vi "MoAgSy_AgentBase.appendData2Variant.vi"(0 "init":variant, 1 "Agent name":string, 2 "journey":string[](array[string]), 3 "Command names":string[](array[string]), 5 "error in":errorcluster, 7 "standard Visitor timeout in ms":i32, 9 "standard visitor":refnum<class "MoAgSy_Visitor.lvclass">) -> (14 "dup init":variant, 19 "error out":errorcluster)   [LabVIEW 2009, in "MoAgSy_Base.lvlib" / "MoAgSy_AgentBase.lvclass"]
doc: "Empty Agent Name:\nKey ID is set as Agent Name"
uses:
  MoAgSy_AgentBase.lvclass
  Visitors/MoAgSy_Visitor/MoAgSy_Visitor.lvclass
  MoAgSy_GPG/MoAgSy_GPG.lvclass
  MoAgSy_Factory/MoAgSy_Factory.lvclass
  HGF_BaseClasses/HGF_Factory/HGF_Factory.lvclass
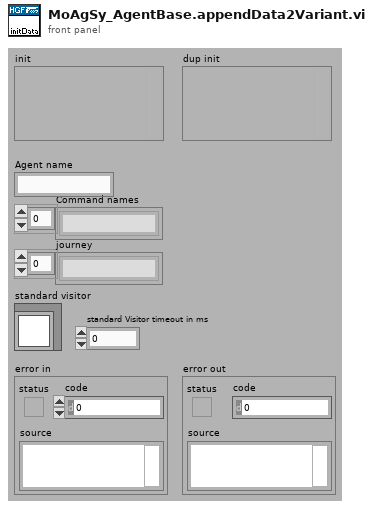
[diagram p1: front panel]
types:
  T1 = cluster{"standard visitor":refnum<class "MoAgSy_Visitor.lvclass">, "standard Visitor timeout in ms":i32}
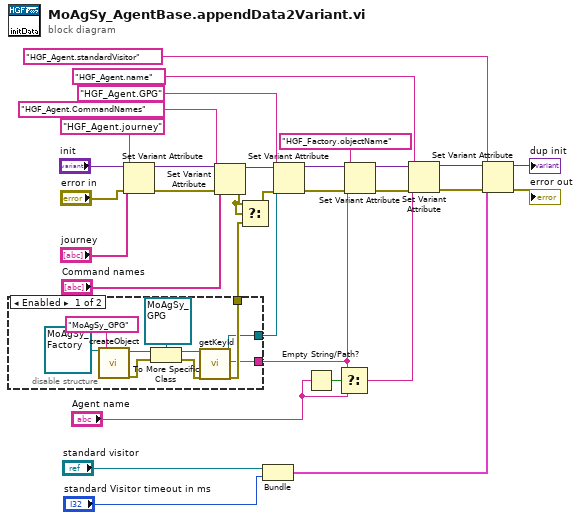
[diagram p0: block diagram]
diagram:
  n1 = disable-structure shown="Enabled" {
    disable-tunnel: [w34 _] -> w22
    disable-tunnel: [w33 _] -> w21
    disable-tunnel: [w32 _] -> w12
    frame #0 {
      n2 = call "createObject.vi"("HGF_Factory"=refnum<class "MoAgSy_Factory.lvclass"> refnum ("MoAgSy.lvlib:MoAgSy_Factory.lvclass"), "className"="MoAgSy_GPG") -> ("HGF_Object"=w39:refnum<class "HGF_Factory.lvclass">, "error out"=w40:errorcluster)  [unwired: 3 in, 13 out]
      n3 = To More Specific Class(target class=refnum<class "MoAgSy_GPG.lvclass"> refnum ("MoAgSy.lvlib:MoAgSy_GPG.lvclass"), reference=w39, error in=w40) -> (specific class reference=w36:refnum<class "MoAgSy_GPG.lvclass">, error out=w35:errorcluster)
      n4 = call-dynamic "getKeyId.vi"("HGF_GPG.lvclass in"=w36, "error in (no error)"=w35) -> ("HGF_GPG.lvclass out"=w33:refnum<class "MoAgSy_GPG.lvclass">, "Key-ID"=w32:string, "error out"=w34:errorcluster)  [unwired: 15 out]
    }
    frame #1 {
    }
  }
  n5 = Set Variant Attribute(Variant="init", name="HGF_Agent.journey", value="journey", error in="error in") -> (Variant out=w30:variant, error out=w28:errorcluster)  [unwired: 1 out]
  n6 = Set Variant Attribute(Variant=w30, name="HGF_Agent.CommandNames", value="Command names", error in=w28) -> (Variant out=w16:variant, error out=w18:errorcluster)  [unwired: 1 out]
  n7 = Select(t=w18, s=w18, f=w22) -> (s? t:f=w17:errorcluster)
  n8 = Bundle("standard visitor"="standard visitor", "standard Visitor timeout in ms"="standard Visitor timeout in ms") -> (w1:T1)  [unwired: 1 in]
  n9 = Set Variant Attribute(Variant=w16, name="HGF_Agent.GPG", value=w21, error in=w17) -> (Variant out=w15:variant, error out=w14:errorcluster)  [unwired: 1 out]
  n10 = Empty String/Path?(string/path="Agent name") -> (empty?=w13:bool)
  n11 = Select(t=w12, s=w13, f="Agent name") -> (s? t:f=w10:string)
  n12 = Set Variant Attribute(Variant=w15, name="HGF_Factory.objectName", value=w12, error in=w14) -> (Variant out=w9:variant, error out=w6:errorcluster)  [unwired: 1 out]
  n13 = Set Variant Attribute(Variant=w9, name="HGF_Agent.name", value=w10) -> (Variant out=w8:variant)  [unwired: 1 in, 2 out]
  n14 = Set Variant Attribute(Variant=w8, name="HGF_Agent.standardVisitor", value=w1, error in=w6) -> (Variant out=→"dup init":variant, error out=→"error out":errorcluster)  [unwired: 1 out]
